vi "Remove Signals.vi"(8 "error in (no error)":errorcluster, 9 "Signal Array":T1[](array[typedef]), 10 "Action":T2, 11 "Custom Device reference in":refnum<k24>) -> (0 "error out":errorcluster, 3 "Custom Device reference out":refnum<k24>)   [LabVIEW 2023, in "J1939 System Definition API Support.lvlib"]
uses:
  J1939 System Definition API Support.lvlib
  NationalInstruments.VeriStand.SystemDefinitionAPI
  Types/Remove Frame Action.ctl
  Types/Remove Item - Frame Cluster.ctl
  Addon/Addon Shared/SubVIs/Constants.vi
  <vilib>/NI VeriStand/Custom Device Tools/Custom Device Utility Library/NI VeriStand - Search for All Items by GUID.vi
  <vilib>/NI VeriStand/Custom Device Tools/Custom Device Utility Library/NI VeriStand - Search for Item by Name.vi
  <vilib>/NI VeriStand/Custom Device Tools/Custom Device Utility Library/Custom Device Utility Library.lvlib
  <vilib>/NI VeriStand/Custom Device API/Custom Device API.lvlib
  Addon/Addon Shared/J1939 Addon Shared.lvlib
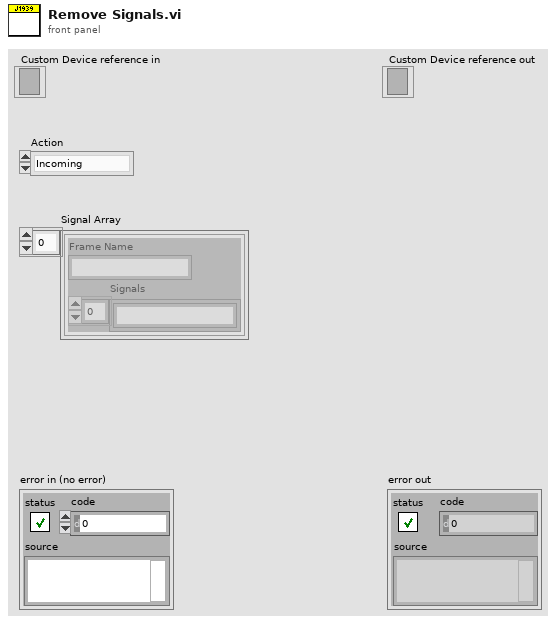
[diagram p1: front panel]
types:
  T1 = typedef "J1939 System Definition API Support.lvlib/Remove Item - Frame Cluster.ctl" = cluster{"Frame Name":string, "Signals":string[]}
  T2 = typedef "J1939 System Definition API Support.lvlib/Remove Frame Action.ctl" = enum16{"Incoming", "Outgoing Event", "Outgoing Cyclic", "Outgoing Cyclic Event"}
  T3 = typedef "Custom Device API.lvlib/Custom Device Item Ref.ctl" = u64
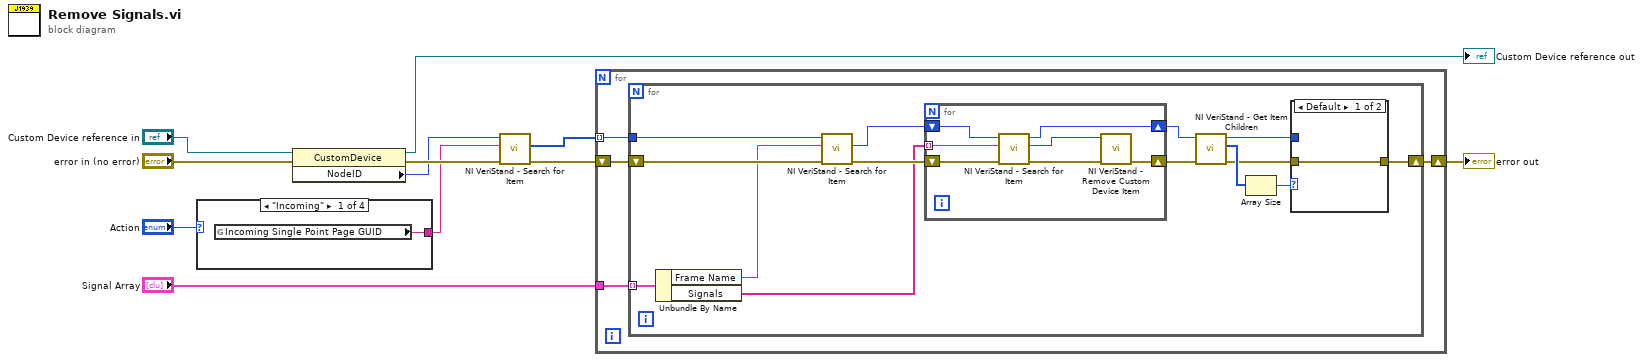
[diagram p0: block diagram]
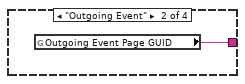
[diagram p2: hidden frame]
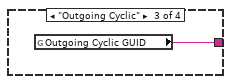
[diagram p3: hidden frame]
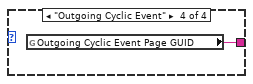
[diagram p4: hidden frame]
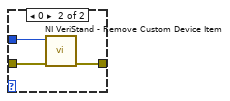
[diagram p5: hidden frame]
diagram:
  n1 = case shown="\"Incoming\"" "Action" {
    tunnel: [w12 w13 w14 w15] -> w1
    frame "Incoming" {
      n2 = global read "Constants.vi" "Incoming Single Point Page GUID"() -> (w12:string)
    }
    frame "Outgoing Event" {
      n3 = global read "Constants.vi" "Outgoing Event Page GUID"() -> (w13:string)
    }
    frame "Outgoing Cyclic" {
      n4 = global read "Constants.vi" "Outgoing Cyclic GUID"() -> (w14:string)
    }
    frame "Outgoing Cyclic Event" {
      n5 = global read "Constants.vi" "Outgoing Cyclic Event Page GUID"() -> (w15:string)
    }
  }
  n6 = property class="CustomDevice"(reference="Custom Device reference in", error in="error in (no error)") -> (reference out=→"Custom Device reference out":refnum<k24>, error out=w8:errorcluster, "NodeID"=w7:u64)
  n7 = call-poly <vilib>:"NI VeriStand - Search for Item.vi"("error in"=w8, "Item GUID"=w1, "Section Ref in"=w7) -> ("error out"=w5:errorcluster, "Item Refs"=w6:T3[])  [unwired: 5 in, 2 out]
  n8 = for {
    tunnel: w6 -> [w19] mode=indexing
    tunnel: "Signal Array" -> [w16]
    shift-right: [w17] -> w4
    shift-left: w5 -> [w18]
    n9 = for {
      tunnel: w19 -> [w33]
      tunnel: w16 -> [w30] mode=indexing
      shift-right: [w23] -> w17
      shift-left: w18 -> [w32]
      n10 = Unbundle By Name(w30) -> ("Frame Name"=w29:string, "Signals"=w28:string[])
      n11 = call-poly <vilib>:"NI VeriStand - Search for Item.vi"("error in"=w32, "Item Name"=w29, "Section Ref in"=w33) -> ("error out"=w31:errorcluster, "Item Ref"=w20:T3)  [unwired: 5 in, 2 out]
      n12 = for {
        shift-right: [w44] -> w26
        shift-left: w31 -> [w43]
        tunnel: w28 -> [w40] mode=indexing
        shift-right: [w38] -> w27
        shift-left: w20 -> [w41]
        n13 = call-poly <vilib>:"NI VeriStand - Search for Item.vi"("error in"=w43, "Item Name"=w40, "Section Ref in"=w41) -> ("error out"=w42:errorcluster, "Item Ref"=w39:T3, "Section Ref out"=w38:T3)  [unwired: 5 in, 1 out]
        n14 = call <vilib>:"NI VeriStand - Remove Custom Device Item.vi"("error in (no error)"=w42, "Item Ref in"=w39) -> ("error out"=w44:errorcluster)  [unwired: 8 in, 1 out]
      }
      n15 = call <vilib>:"NI VeriStand - Get Item Children.vi"("error in (no error)"=w26, "Item Ref in"=w27) -> ("error out"=w24:errorcluster, "Child Refs"=w25:T3[], "Item Ref out"=w21:T3)  [unwired: 6 in, 1 out]
      n16 = Array Size(array=w25) -> (size(s)=w22:i32)
      n17 = case shown="Default" w22 {
        tunnel: w24 -> [w34 w37]
        tunnel: [w34 w36] -> w23
        tunnel: w21 -> [_ w35]
        frame Default {
        }
        frame 0 {
          n18 = call <vilib>:"NI VeriStand - Remove Custom Device Item.vi"("error in (no error)"=w37, "Item Ref in"=w35) -> ("error out"=w36:errorcluster)  [unwired: 8 in, 1 out]
        }
      }
    }
  }
  "error out" <- w4
